vi "CreateNanosecondTimestamp.vi"(11 "current time":timestamp) -> (3 "Time in RFC3339Nano":dbl)   [LabVIEW 2017, in "hse-logger.lvlib" / "LokiHandler.lvclass"]
doc: "Excerpt from official documentation on how they are interpreted:\n\nThe API accepts several formats for timestamps. An integer with ten or fewer digits is interpreted as a Unix timestamp in seconds. More than ten digits are interpreted as a Unix timestamp in nanoseconds. A floating point number is a Unix timestamp with fractions of a second.\n\nThe timestamps can also be written in RFC3339 and RFC3339Nano format, as supported by Go’s time package."
uses:
  LokiHandler.lvclass
  LokiHandler.lvclass/LokiHandler.ctl
panel:
  # "Connector Pane"
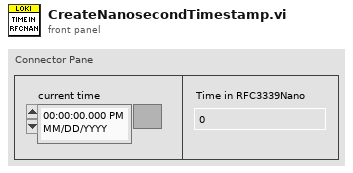
[diagram p1: front panel]
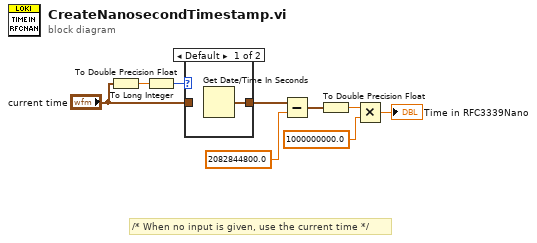
[diagram p0: block diagram]
diagram:
  # "/* When no input is given, use the current time */"
  n1 = To Double Precision Float(number="current time") -> (double precision float=w9:dbl)
  n2 = To Long Integer(number=w9) -> (32bit integer=w8:i32)
  n3 = case shown="Default" w8 {
    tunnel: [w10 w11] -> w2
    tunnel: "current time" -> [_ w11]
    frame Default {
      n4 = Get Date/Time In Seconds() -> (seconds since 1Jan1904=w10:timestamp)
    }
    frame 0 {
    }
  }
  n5 = Subtract(x=w2, y=2082844800.0) -> (x-y=w5:timestamp)
  n6 = To Double Precision Float(number=w5) -> (double precision float=w6:dbl)
  n7 = Multiply(x=w6, y=1000000000.0) -> (x*y=→"Time in RFC3339Nano":dbl)
